vi "HEWH Error Handler.vi"(0 "Equipment":T2={"COM Port"="COM5", "MW100"="MW100", "AG34970"="A-34972A", "Chamber"="WT500"}, 1 "MW100 Semiphore":T1, 2 "file path":path=path "c:/work/errorlog.txt", 11 "error in (no error)":errorcluster) -> (15 "Error Out (no error)":errorcluster)   [LabVIEW 2012]
uses:
  EquipReferences.ctl
  <vilib>/Utility/file.llb/Write To Spreadsheet File (string).vi
  Drivers/Agilent 34970/Agilent 34970.lvlib
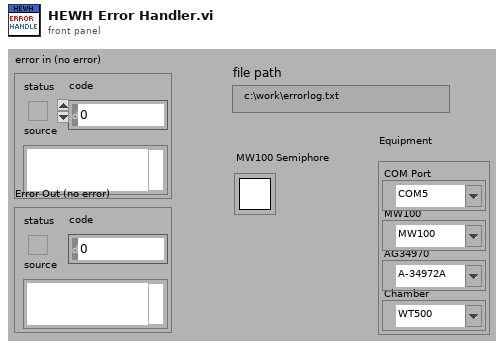
[diagram p1: front panel]
types:
  T1 = typedef "Semaphore RefNum" = refnum<k1>
  T2 = typedef "EquipReferences.ctl" = cluster{"COM Port":refnum<visa-resource-name>, "MW100":refnum<visa-resource-name>, "AG34970":refnum<visa-resource-name>, "Chamber":refnum<visa-resource-name>}
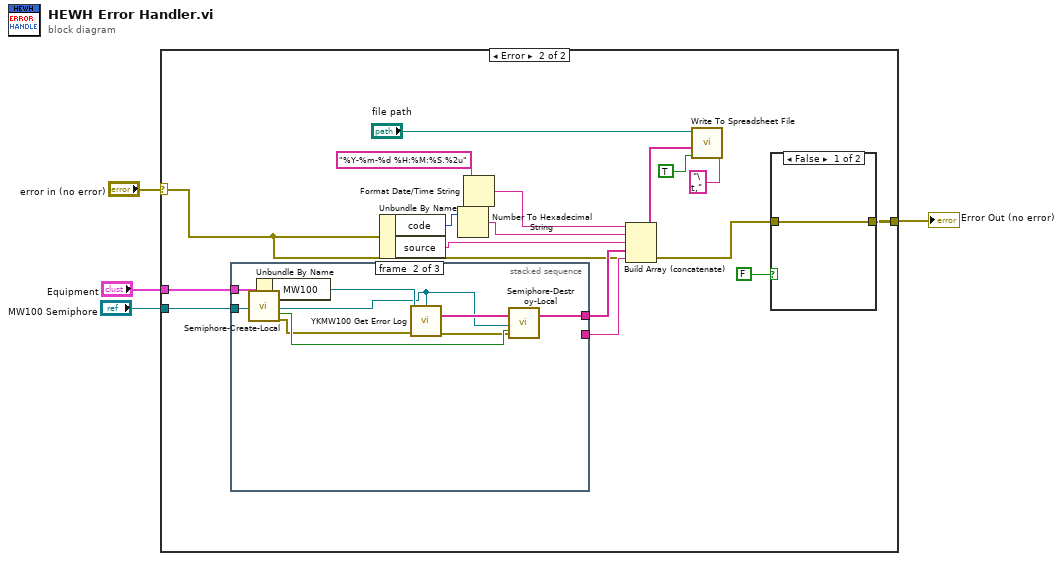
[diagram p0: block diagram]
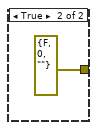
[diagram p3: hidden frame]
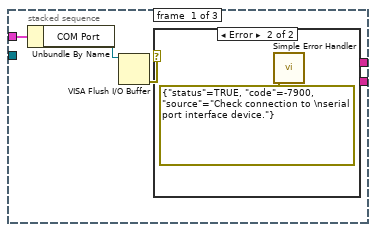
[diagram p4: hidden frame]
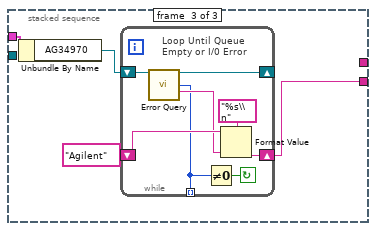
[diagram p6: hidden frame]
diagram:
  n1 = case shown="Error" "error in (no error)" {
    selector: "error in (no error)" -> [w5 w6]
    tunnel: [w5 w13] -> w3
    tunnel: "Equipment" -> [_ w12]
    tunnel: "MW100 Semiphore" -> [_ w9]
    frame No Error {
    }
    frame Error {
      n2 = stacked-sequence {
        tunnel: w12 -> [w26 w35 w39]
        tunnel: [_ w33 _] -> w11
        tunnel: [_ _ w36] -> w10
        tunnel: w9 -> [_ w32 _]
        frame #0 {
          n3 = Unbundle By Name(w26) -> ("COM Port"=w25:refnum<visa-resource-name>)
          n4 = VISA Flush I/O Buffer(VISA resource name=w25) -> (error out=w24:errorcluster)  [unwired: 2 in, 1 out]
          n5 = case shown="Error" w24 {
            frame No Error {
            }
            frame Error {
              n6 = call <vilib>:"Simple Error Handler.vi"("error in (no error)"=errorcluster {"status"=TRUE, "code"=-7900, "source"="Check connection to \nserial port interface device."}) -> ()  [unwired: 4 in, 5 out]
            }
          }
        }
        frame #1 {
          n7 = call "Semiphore-Create-Local.vi"("Semiphore"=w32) -> ("semaphore"=w28:T1, "Local?"=w31:bool, "error out"=w30:errorcluster)  [unwired: 16 in]
          n8 = Unbundle By Name(w35) -> ("MW100"=w34:refnum<visa-resource-name>)
          n9 = call "YKMW100 Get Error Log.vi"("VISA session"=w34, "Semiphore"=w28, "error in (no error)"=w30) -> ("Error History"=w33:string[], "error out"=w29:errorcluster)  [unwired: 9 in, 2 out]
          n10 = call "Semiphore-Destroy-Local.vi"("Semiphore"=w28, "Local?"=w31, "error in (no error)"=w29) -> ()  [unwired: 16 in, 1 out]
        }
        frame #2 {
          n11 = Unbundle By Name(w39) -> ("AG34970"=w38:refnum<visa-resource-name>)
          n12 = while {
            tunnel: [w41] -> _ mode=indexing
            shift-left: w38 -> [w40]
            shift-right: [w47] -> _
            shift-left: "Agilent" ("output string") -> [w44]
            shift-right: [w46] -> w36
            stop <- w42 continue-if-true
            # "Loop Until Queue Empty or I/0 Error"
            n13 = call "Error Query.vi"("VISA Resource Name"=w40) -> ("VISA Resource Name Out"=w47:refnum<visa-resource-name>, "Error"=w41:i32, "Error Message"=w43:string)  [unwired: 11 in, 1 out]
            n14 = Not Equal To 0?(x=w41) -> (x != 0?=w42:bool)
            n15 = Format Value(string ("")=w44, format string="%s\\n", value (0)=w43) -> (output string=w46:string)
          }
        }
      }
      n16 = Unbundle By Name(w6) -> ("code"=w17:i32, "source"=w18:string)
      n17 = Number To Hexadecimal String(2:w17) -> (0:w16:string)  [unwired: 1 in]
      n18 = Format Date/Time String(time format string (%c)="%Y-%m-%d %H:%M:%S.%2u") -> (date/time string=w15:string)  [unwired: 2 out]
      n19 = Build Array (concatenate)(w15, w16, w18, w11, w10) -> (w14:string[])
      n20 = call-poly <vilib>:"Write To Spreadsheet File.vi"("delimiter (\\t)"="\t," ("delimiter (\\t)"), "append to file? (new file:F)"=TRUE, "1D data"=w14, "file path (dialog if empty)"="file path") -> ()  [unwired: 4 in, 1 out]
      n21 = case shown="False" FALSE {
        tunnel: [w22 errorcluster {"status"=FALSE, "code"=0, "source"=""} ("Error Out (no error)")] -> w13
        tunnel: w6 -> [w22 _]
        frame False {
        }
        frame True {
        }
      }
    }
  }
  "Error Out (no error)" <- w3
